vi "RH_DCPower_UpdateConfiguration.vi"(7 "DCPower_Parameters":T1={"Output"=enum."DC Voltage", "Current_range"=0.0, "Current"=0.0, "Voltage_range"=0.0, "Voltage"=0.0, "Aperture_time"=0.0, "Source Delay"=0.0, "Sense"=1008} {"Source Delay" format="%.6p"; "Sense" items=["Local"=1008, "Remote"=1009]; "Aperture_time" format="%.6p"; "Current_range" format="%.6p"; "Current" format="%.6p"; "Voltage_range" format="%.6p"; "Voltage" format="%.6p"}, 8 "error in (no error)":errorcluster, 10 "channel name":string, 11 "DCPower Session In":refnum<k15>) -> (0 "error out":errorcluster, 3 "DCPower Session Out":refnum<k15>)   [LabVIEW 2023, in "ResourceHandling.lvlib"]
doc: "Update Configuration to DC Voltage or DC Current mode"
uses:
  ResourceHandling.lvlib
  TypeDefs/RH_DCPower_Parameters.ctl
  <instrlib>/niDCPower/nidcpower.llb/niDCPower Output Function.ctl
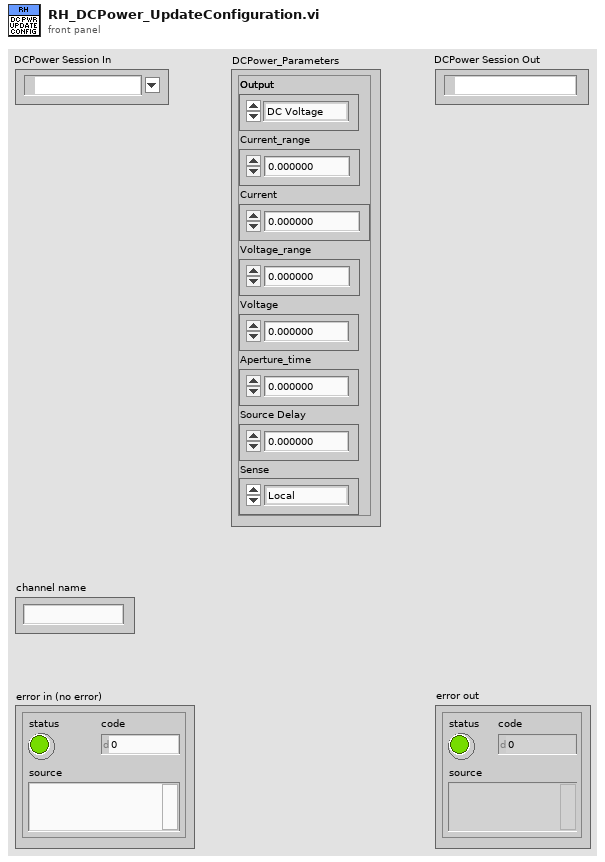
[diagram p1: front panel]
types:
  T1 = typedef "ResourceHandling.lvlib/RH_DCPower_Parameters.ctl" = cluster{"Output":enum16{"DC Voltage", "DC Current"}, "Current_range":dbl, "Current":dbl, "Voltage_range":dbl, "Voltage":dbl, "Aperture_time":dbl, "Source Delay":dbl, "Sense":i32}
  T2 = typedef "niDCPower Output Function.ctl" = i32
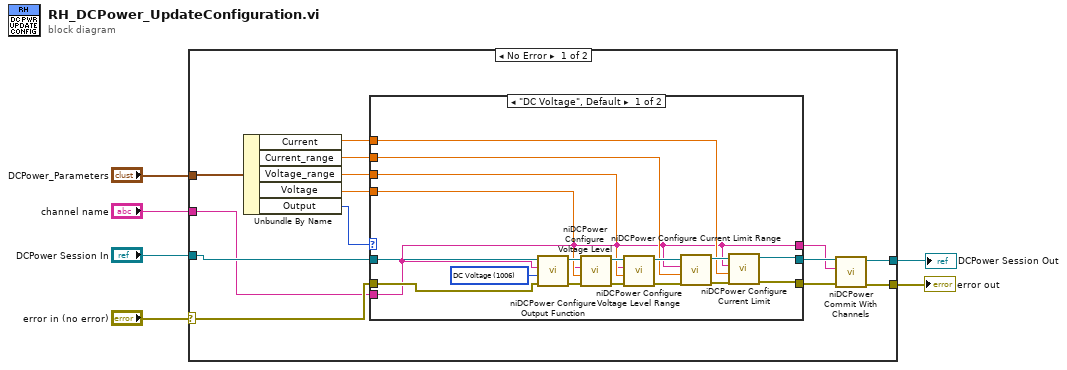
[diagram p0: block diagram]
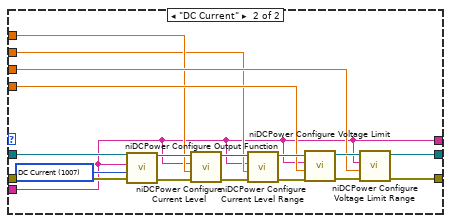
[diagram p2: hidden frame]
diagram:
  n1 = case shown="No Error" "error in (no error)" {
    selector: "error in (no error)" -> [w12 w58]
    tunnel: "DCPower_Parameters" -> [w16 _]
    tunnel: "DCPower Session In" -> [w15 w57]
    tunnel: [w14 w57] -> w1
    tunnel: [w13 w58] -> w5
    tunnel: "channel name" -> [w7 _]
    frame No Error {
      n2 = Unbundle By Name(w16) -> ("Current"=w17:dbl, "Current_range"=w18:dbl, "Voltage_range"=w19:dbl, "Voltage"=w20:dbl, "Output"=w11:enum16{"DC Voltage", "DC Current"})
      n3 = case shown="\"DC Voltage\", Default" w11 {
        tunnel: w12 -> [w30 w48]
        tunnel: w15 -> [w31 w47]
        tunnel: [w24 w43] -> w10
        tunnel: [w23 w42] -> w9
        tunnel: w20 -> [w33 w44]
        tunnel: w19 -> [w32 w45]
        tunnel: w18 -> [w27 w40]
        tunnel: w17 -> [w22 w41]
        tunnel: w7 -> [w21 w39]
        tunnel: [w21 w39] -> w8
        frame "DC Voltage", Default {
          w34 = T2 1006 items=["DC Voltage"=1006, "DC Current"=1007, "Pulse Voltage"=1049, "Pulse Current"=1050] ("output function")
          n4 = call <instrlib>:"niDCPower Configure Output Function.vi"("error in (no error)"=w30, "output function"=w34, "channel name"=w21, "instrument handle"=w31) -> ("error out"=w36:errorcluster, "instrument handle out"=w35:refnum<k15>)  [unwired: 6 in]
          n5 = call <instrlib>:"niDCPower Configure Voltage Level.vi"("error in (no error)"=w36, "voltage level"=w33, "channel name"=w21, "instrument handle"=w35) -> ("error out"=w38:errorcluster, "instrument handle out"=w37:refnum<k15>)  [unwired: 6 in]
          n6 = call <instrlib>:"niDCPower Configure Voltage Level Range.vi"("error in (no error)"=w38, "voltage level range"=w32, "channel name"=w21, "instrument handle"=w37) -> ("error out"=w29:errorcluster, "instrument handle out"=w28:refnum<k15>)  [unwired: 6 in]
          n7 = call <instrlib>:"niDCPower Configure Current Limit Range.vi"("error in (no error)"=w29, "current limit range"=w27, "channel name"=w21, "instrument handle"=w28) -> ("error out"=w26:errorcluster, "instrument handle out"=w25:refnum<k15>)  [unwired: 6 in]
          n8 = call <instrlib>:"niDCPower Configure Current Limit.vi"("error in (no error)"=w26, "current limit"=w22, "channel name"=w21, "instrument handle"=w25) -> ("error out"=w23:errorcluster, "instrument handle out"=w24:refnum<k15>)  [unwired: 6 in]
        }
        frame "DC Current" {
          w46 = T2 1007 items=["DC Voltage"=1006, "DC Current"=1007, "Pulse Voltage"=1049, "Pulse Current"=1050] ("output function")
          n9 = call <instrlib>:"niDCPower Configure Output Function.vi"("error in (no error)"=w48, "output function"=w46, "channel name"=w39, "instrument handle"=w47) -> ("error out"=w49:errorcluster, "instrument handle out"=w50:refnum<k15>)  [unwired: 6 in]
          n10 = call <instrlib>:"niDCPower Configure Current Level.vi"("error in (no error)"=w49, "current level"=w41, "channel name"=w39, "instrument handle"=w50) -> ("error out"=w56:errorcluster, "instrument handle out"=w55:refnum<k15>)  [unwired: 6 in]
          n11 = call <instrlib>:"niDCPower Configure Current Level Range.vi"("error in (no error)"=w56, "current level range"=w40, "channel name"=w39, "instrument handle"=w55) -> ("error out"=w54:errorcluster, "instrument handle out"=w53:refnum<k15>)  [unwired: 6 in]
          n12 = call <instrlib>:"niDCPower Configure Voltage Limit.vi"("error in (no error)"=w54, "voltage limit"=w44, "channel name"=w39, "instrument handle"=w53) -> ("error out"=w52:errorcluster, "instrument handle out"=w51:refnum<k15>)  [unwired: 6 in]
          n13 = call <instrlib>:"niDCPower Configure Voltage Limit Range.vi"("error in (no error)"=w52, "voltage limit range"=w45, "channel name"=w39, "instrument handle"=w51) -> ("error out"=w42:errorcluster, "instrument handle out"=w43:refnum<k15>)  [unwired: 6 in]
        }
      }
      n14 = call <instrlib>:"niDCPower Commit With Channels.vi"("error in (no error)"=w9, "channel name"=w8, "instrument handle"=w10) -> ("error out"=w13:errorcluster, "instrument handle out"=w14:refnum<k15>)  [unwired: 7 in]
    }
    frame Error {
    }
  }
  "error out" <- w5
  "DCPower Session Out" <- w1
